vi "Get State.vi"(8 "error in (no error)":errorcluster, 11 "Pulse Controller in":refnum<class "Pulse Recorder.lvclass">) -> (0 "error out":errorcluster, 1 "Result ready":bool, 2 "Armed":bool, 3 "Pulse Controller out":refnum<class "Pulse Recorder.lvclass">, 4 "Check again":bool)   [LabVIEW 2016, in "Pulse Recorder.lvclass"]
uses:
  Pulse Recorder.lvclass
  C:/github/LabActor/Template Module/Template Module.lvclass
  Pulse Recorder.lvclass/Pulse Recorder.ctl
  Template Module/Template Module.lvclass/Template Module.ctl
  Template Module Messages/Self-Addressed Msg/Self-addressed Msg.lvclass/Self-addressed Msg.ctl
  Controllers/Pulse Controller Messages/Armed Response Msg/Armed Response Msg.lvclass/Armed Response Msg.ctl
  <vilib>/ActorFramework/Message Enqueuer/Message Enqueuer.lvclass/Message Enqueuer.ctl
  Template Module/Read Name.vi
  Template Module/Read Reply to.vi
  Template Module Messages/Self-Addressed Msg/Read Return Enqueuer.vi
  <vilib>/ActorFramework/Message Enqueuer/Enqueue.vi
  Template Module Messages/Result Reply Msg/Result Reply Msg.lvclass
  C:/github/LabActor/Template Module Messages/Self-Addressed Msg/Self-addressed Msg.lvclass
  Controllers/Pulse Controller Messages/Armed Response Msg/Armed Response Msg.lvclass
  C:/Program Files (x86)/National Instruments/LabVIEW 2016/vi.lib/ActorFramework/Message/Message.lvclass
  <vilib>/ActorFramework/Message Priority Queue/Priority Enqueue.vi
  <vilib>/ActorFramework/Message Enqueuer/Message Enqueuer.lvclass
  Instrument Actor/Instrument Actor.lvclass
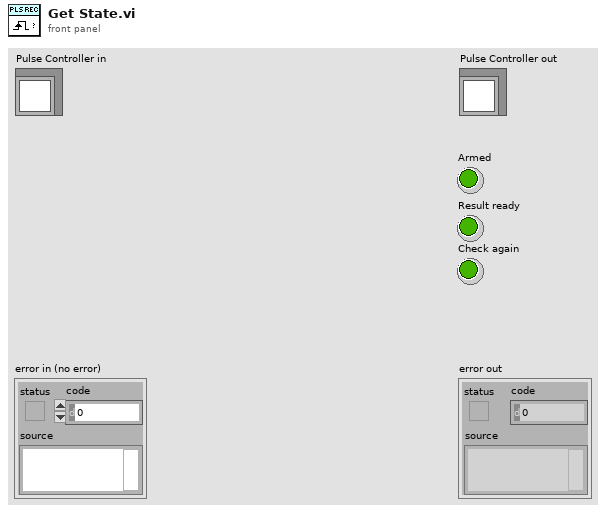
[diagram p1: front panel]
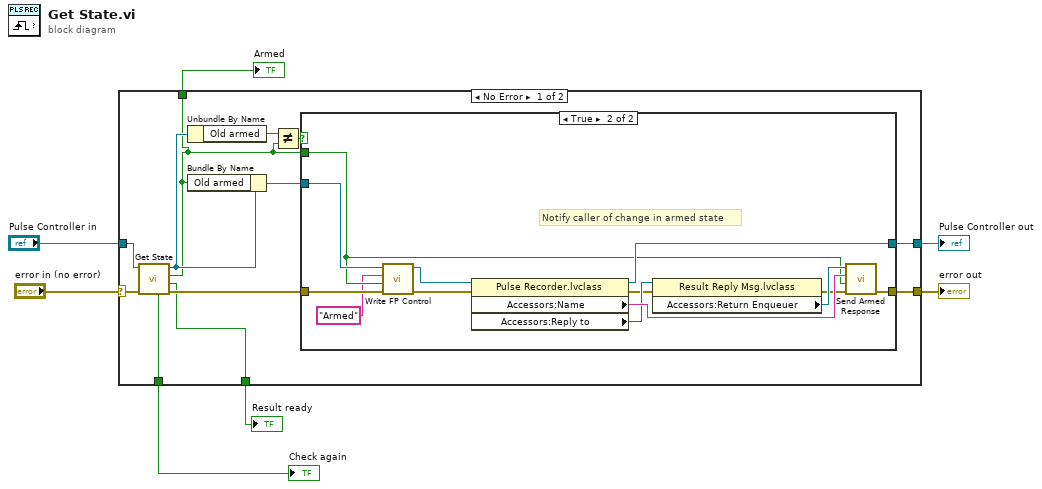
[diagram p0: block diagram]
diagram:
  n1 = case shown="No Error" "error in (no error)" {
    selector: "error in (no error)" -> [w15 w36]
    tunnel: [w16 w36] -> w6
    tunnel: [w12 w35] -> w4
    tunnel: "Pulse Controller in" -> [w14 w35]
    tunnel: [w10 _] -> w3
    tunnel: [w9 _] -> w2
    tunnel: [w8 _] -> w1
    frame No Error {
      n2 = call-parent "Get State.vi"("error in (no error)"=w15, "Instrument Actor in"=w14) -> ("error out"=w11:errorcluster, "Result ready"=w9:bool, "Armed"=w8:bool, "Instrument Actor out"=w13:refnum<class "Pulse Recorder.lvclass">, "Check again"=w10:bool)  [unwired: 5 in]
      n3 = Unbundle By Name(w13) -> ("Old armed"=w19:bool)
      n4 = Bundle By Name(cluster=w13, "Old armed"=w8) -> (w17:refnum<class "Pulse Recorder.lvclass">)
      n5 = Not Equal?(x=w19, y=w8) -> (x != y?=w18:bool)
      n6 = case shown="True" w18 {
        tunnel: w17 -> [w20 w25]
        tunnel: w11 -> [w21 w27]
        tunnel: [w21 w33] -> w16
        tunnel: w8 -> [_ w23]
        tunnel: [w20 w32] -> w12
        frame False {
        }
        frame True {
          # "Notify caller of change in armed state"
          n7 = call-dynamic "Write FP Control.vi"("error in (no error)"=w27, "Control Value"=w23, "Control Name"="Armed", "Measure Object in"=w25) -> ("error out"=w26:errorcluster, "Measure Object out"=w24:refnum<class "Pulse Recorder.lvclass">)  [unwired: 6 in]
          n8 = property class="Pulse Recorder.lvclass"(reference=w24, error in=w26) -> (reference out=w32:refnum<class "Pulse Recorder.lvclass">, error out=w28:errorcluster, "Accessors:Name"=w34:string, "Accessors:Reply to"=w31:refnum<class "Result Reply Msg.lvclass">)
          n9 = property class="Result Reply Msg.lvclass"(reference=w31, error in=w28) -> (error out=w29:errorcluster, "Accessors:Return Enqueuer"=w30:refnum<class "Message Enqueuer.lvclass">)  [unwired: 1 out]
          n10 = call "Send Armed Response.vi"("error in (no error)"=w29, "Armed"=w23, "Sender"=w34, "Message Enqueuer"=w30) -> ("error out"=w33:errorcluster)  [unwired: 6 in, 1 out]
        }
      }
    }
    frame Error {
    }
  }
  "error out" <- w6
  "Pulse Controller out" <- w4
  "Check again" <- w3
  "Result ready" <- w2
  "Armed" <- w1
